vi "Configure Power.vi"(0 "VISA resource name":refnum<visa-resource-name>, 1 "Enable Auto Attenuation (T: Enable)":bool=TRUE, 2 "Enable RF Power (T: Enable)":bool=TRUE, 3 "Enable Power Slope (F: Disable)":bool, 5 "Channel (1)":i32=1, 7 "Port (1)":i32=1, 9 "Attenuation (0 dB)":dbl, 11 "error in (no error)":errorcluster, 12 "Power Level (0 dBm)":dbl, 13 "Power Slope (0 dB/GHz)":dbl) -> (4 "VISA resource name out":refnum<visa-resource-name>, 15 "error out":errorcluster)   [LabVIEW 2018, in "Keysight PNA Series.lvlib"]
doc: "Configures the RF power."
uses:
  Keysight PNA Series.lvlib
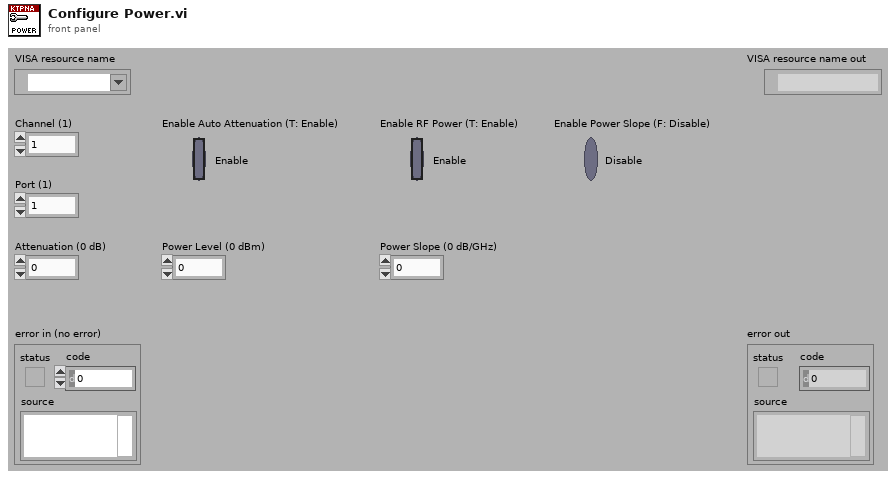
[diagram p1: front panel]
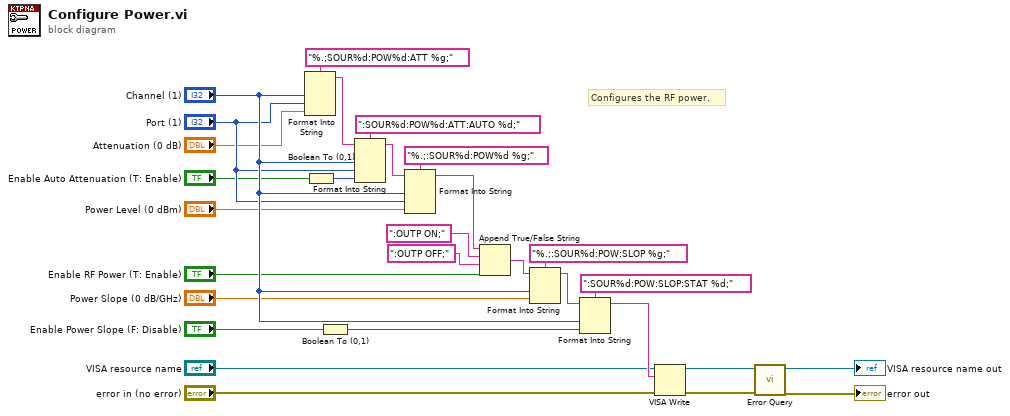
[diagram p0: block diagram]
diagram:
  # "Configures the RF power."
  n1 = Format Into String(format string="%.;SOUR%d:POW%d:ATT %g;", "Channel (1)", "Port (1)", "Attenuation (0 dB)") -> (resulting string=w25:string)  [unwired: 2 in, 1 out]
  n2 = Boolean To (0,1)(Boolean="Enable Auto Attenuation (T: Enable)") -> (0, 1=w3:i16)
  n3 = Boolean To (0,1)(Boolean="Enable Power Slope (F: Disable)") -> (0, 1=w1:i16)
  n4 = Format Into String(format string=":SOUR%d:POW%d:ATT:AUTO %d;", initial string=w25, "Channel (1)", "Port (1)", w3) -> (resulting string=w23:string)  [unwired: 1 in, 1 out]
  n5 = Format Into String(format string="%.;:SOUR%d:POW%d %g;", initial string=w23, "Channel (1)", "Port (1)", "Power Level (0 dBm)") -> (resulting string=w20:string)  [unwired: 1 in, 1 out]
  n6 = Append True/False String(1:"Enable RF Power (T: Enable)", 2:":OUTP OFF;", 3:":OUTP ON;", 4:w20) -> (0:w16:string)
  n7 = Format Into String(format string="%.;:SOUR%d:POW:SLOP %g;", initial string=w16, "Channel (1)", "Power Slope (0 dB/GHz)") -> (resulting string=w13:string)  [unwired: 1 in, 1 out]
  n8 = Format Into String(format string=":SOUR%d:POW:SLOP:STAT %d;", initial string=w13, "Channel (1)", w1) -> (resulting string=w11:string)  [unwired: 1 in, 1 out]
  n9 = VISA Write(VISA resource name="VISA resource name", write buffer=w11, error in (no error)="error in (no error)") -> (VISA resource name out=w8:refnum<visa-resource-name>, error out=w7:errorcluster)  [unwired: 1 out]
  n10 = call "Error Query.vi"("error in (no error)"=w7, "VISA resource name"=w8) -> ("error out"=→"error out":errorcluster, "VISA resource name out"=→"VISA resource name out":refnum<visa-resource-name>)  [unwired: 6 in, 2 out]
